vi "Video feed info class VI - change beginning-end cursor states.vi"(8 "error in (no error)":errorcluster, 9 "Higher Cursor value":u32, 10 "Lower Cursor value":u32, 11 "Video feed info in":refnum<class "Video feed info.lvclass">) -> (0 "error out":errorcluster, 3 "Video feed info out":refnum<class "Video feed info.lvclass">)   [LabVIEW 2010, in "Video feed info.lvclass"]
uses:
  Video feed info.lvclass
  Video feed info.lvclass/Video feed info.ctl
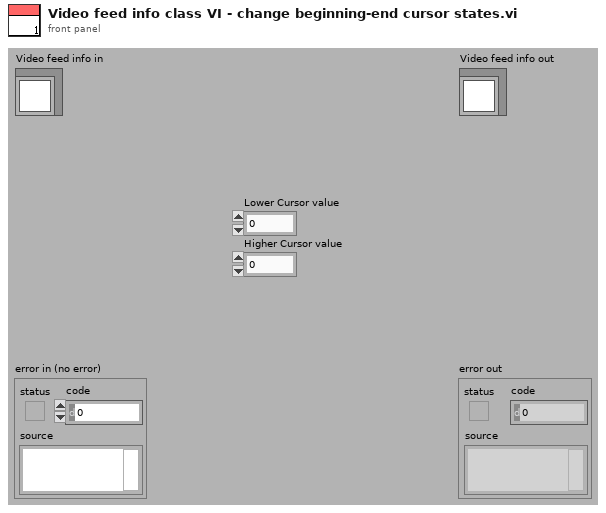
[diagram p1: front panel]
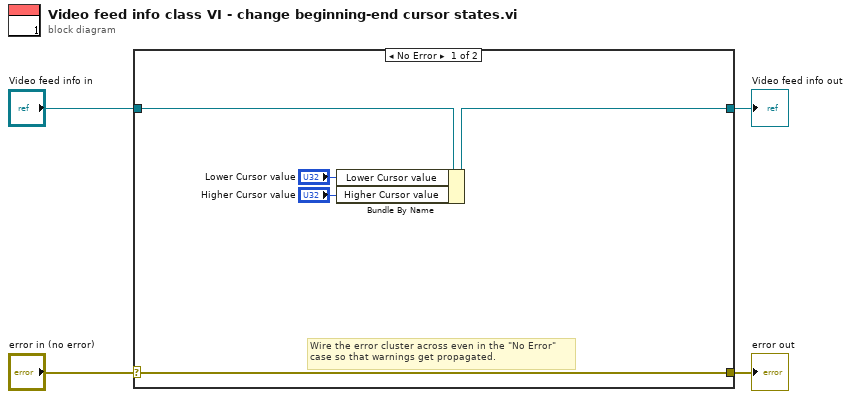
[diagram p0: block diagram]
diagram:
  n1 = case shown="No Error" "error in (no error)" {
    selector: "error in (no error)" -> [w8 w11]
    tunnel: [w8 w11] -> w3
    tunnel: [w7 w10] -> w1
    tunnel: "Video feed info in" -> [w9 w10]
    frame No Error {
      # "Wire the error cluster across even in the \"No Error\"\ncase so that warnings get propagated."
      n2 = Bundle By Name(cluster=w9, "Lower Cursor value"="Lower Cursor value", "Higher Cursor value"="Higher Cursor value") -> (w7:refnum<class "Video feed info.lvclass">)
    }
    frame Error {
    }
  }
  "error out" <- w3
  "Video feed info out" <- w1
